vi "Host.vi"() -> ()   [LabVIEW 2022 SP3]
uses:
  <vilib>/FPGAPlugInAG/PXIe-7972R/niLvFpga_Open_PXIe-7972R.vi
  <vilib>/rvi/interface/common/dynamic/niFpgaDynamicAddResources.vi
  <vilib>/Utility/error.llb/Error Cluster From Error Code.vi
  <vilib>/rvi/errors/niLvFpgaAdjustHostInterfaceError.vi
  <vilib>/FPGAPlugInAG/Dynamic/niLvFpga_Close_Dynamic.vi
  <vilib>/rvi/interface/nirviOpenFPGA/nirviOpenFPGA.xnode
  FPGA Bitfiles/untitledproject1_FPGATarget_7972RFPGAVIfirst_8hhnNsn05bY.lvbitx
  <vilib>/rvi/interface/nirviMethod/nirviMethod.xnode
  <vilib>/rvi/interface/nirviReadWriteControl/nirviReadWriteControl.xnode
  <vilib>/rvi/interface/nirviCloseFPGA/nirviCloseFPGA.xnode
  <vilib>/FPGAPlugInAG/Dynamic/niLvFpga_ReadFifo_Dynamic.vi
  <vilib>/rvi/errors/niLvFpgaMergeErrorWithErrorCode.vi
  NiFpgaLv.dll
  <vilib>/rvi/interface/Simulation/niFpgaSimulationCallBeginRW.vi
panel:
  out "Genarated\nSignal":waveform(i16)(graph)
  in  "Number of Elements":u32
  in  "White Noise Amplitude":u16
  out "X":waveform(i16)(graph)
  in  "Sine Frequency":dbl
  in  "Add white noise?":bool
  in  "Signal Generator\nSelect":enum16{"Square", "Sawtooth", "Sine"}(ring)
  out "AI 1 - Filtered 2":waveform(dbl)(graph)
  in  "DMA FIFO Resolution":u32
  in  "Sawtooth Frequency":i16
  in  "Square Frequency":i16
  out "Y":waveform(i16)(graph)
  out "AI 1 - Raw":waveform(dbl)(graph)
  in  "stop":bool
  out "error out":errorcluster
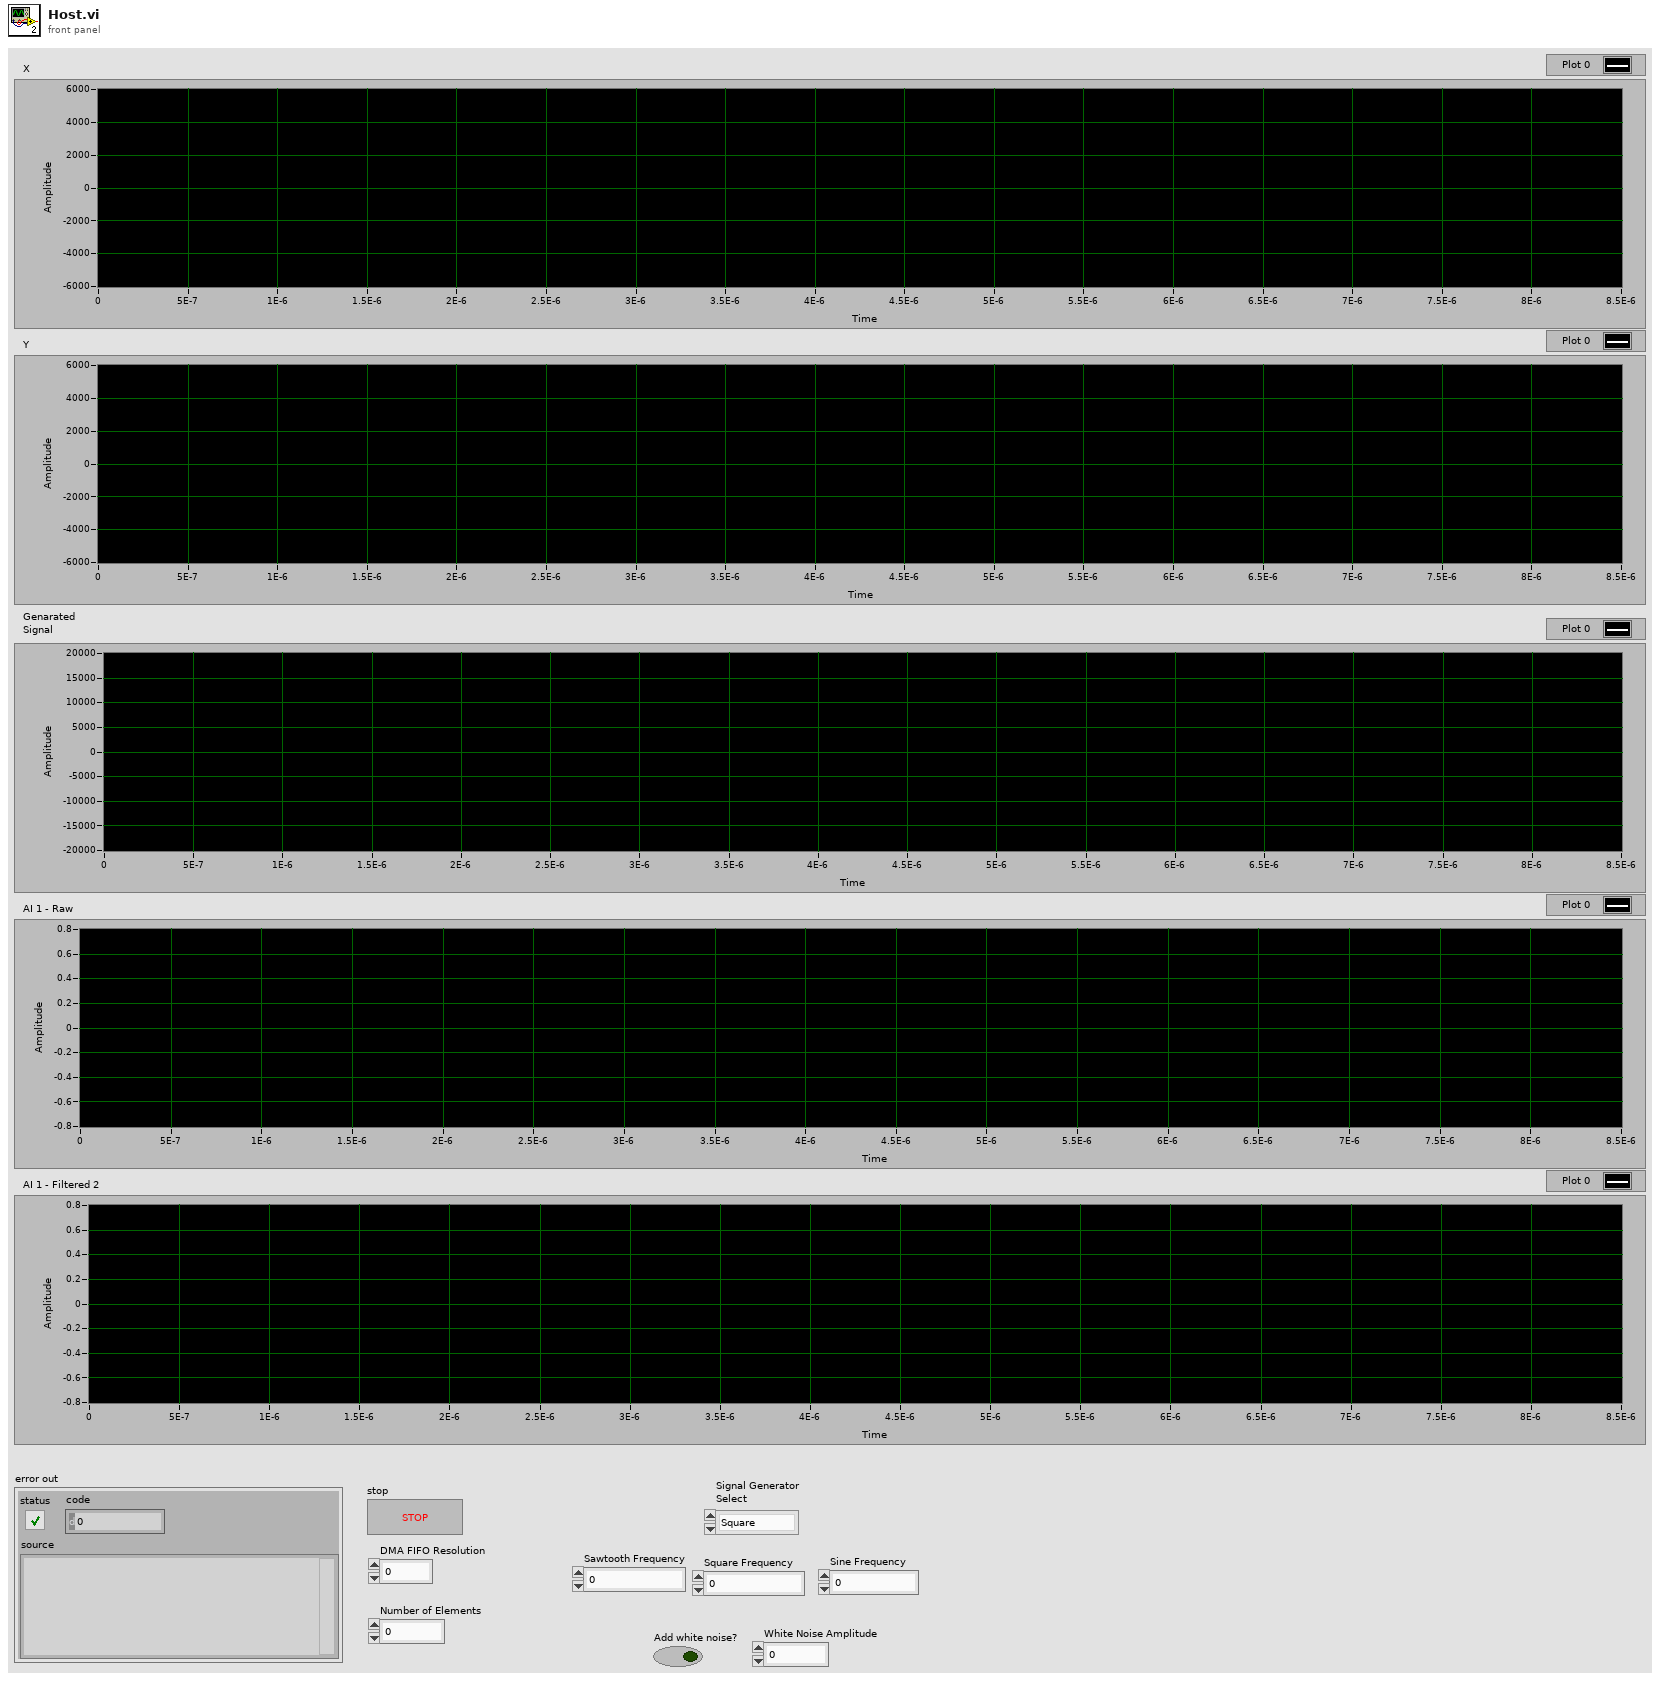
[diagram p1: front panel]
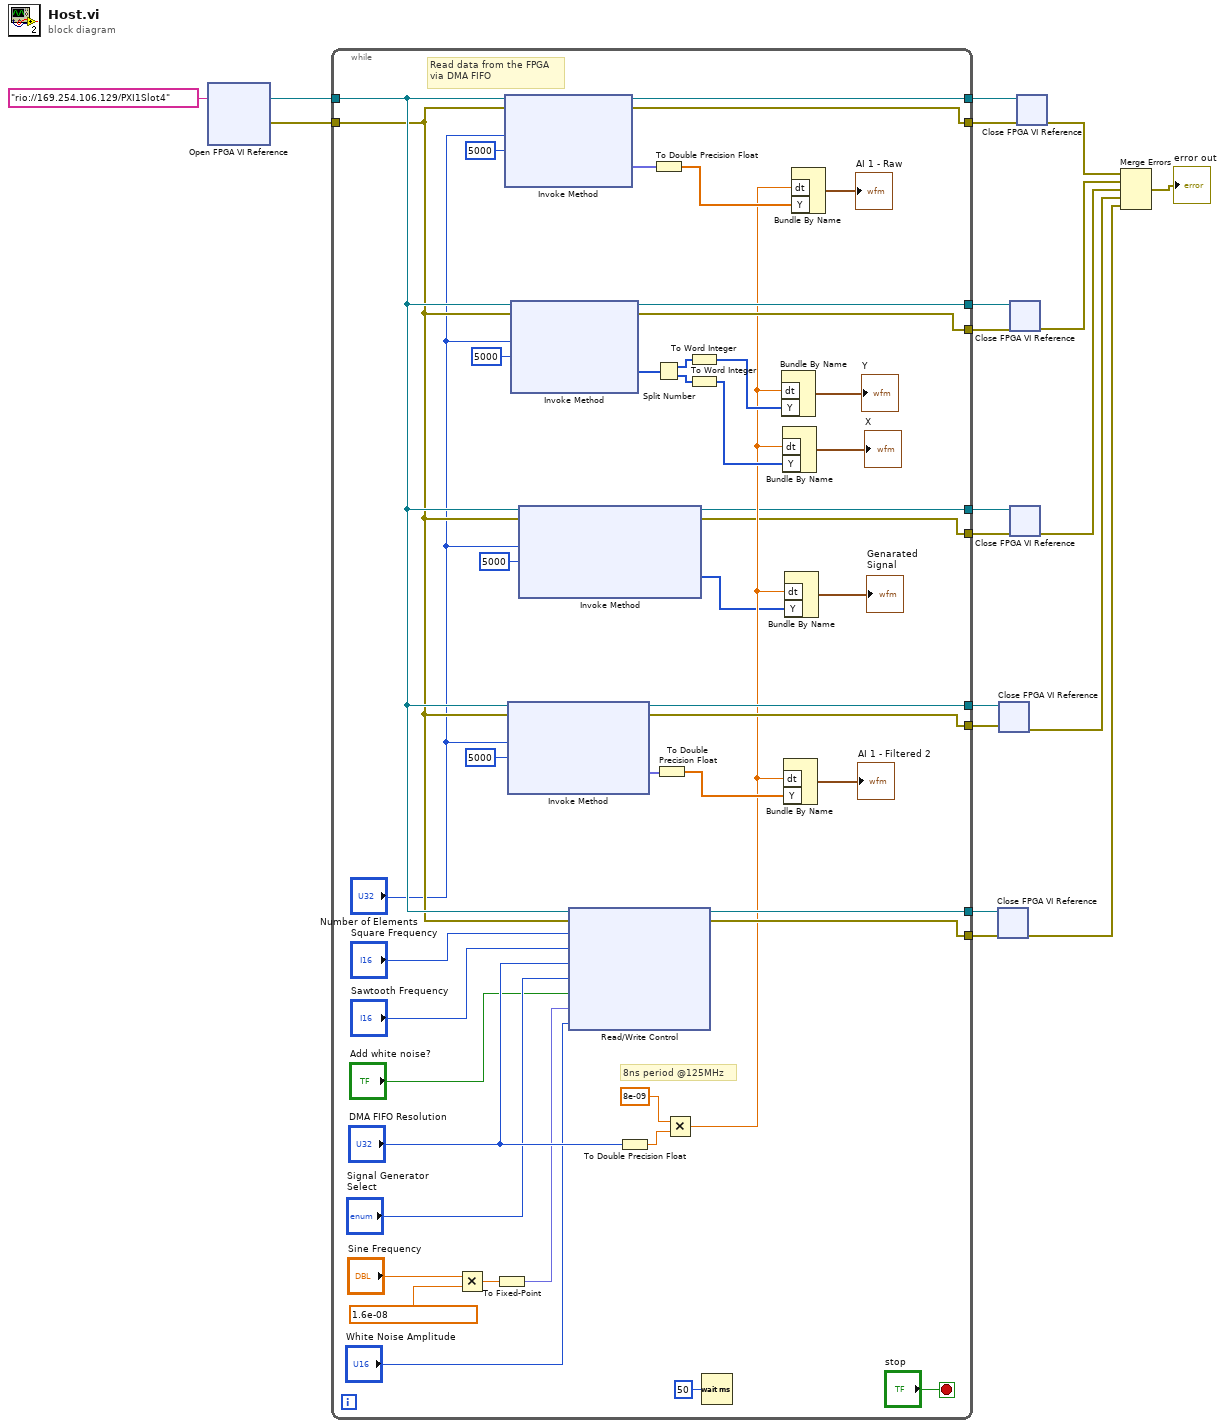
[diagram p0: block diagram]
diagram:
  n1 = xnode "Open FPGA VI Reference"("resource name"=tag "rio://169.254.106.129/PXI1Slot4") -> ("FPGA VI Reference Out"=w18:refnum<k20>, "error out"=w17:errorcluster)  [unwired: 1 in]
  n2 = while {
    tunnel: w18 -> [w27]
    tunnel: w17 -> [w26]
    tunnel: [w63] -> w16
    tunnel: [w60] -> w15
    tunnel: [w59] -> w12
    tunnel: [w57] -> w14
    tunnel: [w58] -> w10
    tunnel: [w30] -> w8
    tunnel: [w48] -> w7
    tunnel: [w47] -> w6
    tunnel: [w22] -> w3
    tunnel: [w21] -> w2
    stop <- "stop" stop-if-true
    # "Read data from the FPGA\nvia DMA FIFO"
    # "8ns period @125MHz"
    n3 = Multiply(x="Sine Frequency", y=1.6e-08 ("delta_t")) -> (x*y=w43:dbl)
    n4 = To Fixed-Point(number=w43) -> (fixed-point=w39:fxp<+/-,64,4>)  [unwired: 1 in]
    n5 = xnode "Invoke Method"("FPGA VI Reference In"=w27, "error in"=w26, "Number of Elements"="Number of Elements", "Timeout (ms)"=5000) -> ("FPGA VI Reference Out"=w63:refnum<k20>, "error out"=w59:errorcluster, "Data"=w62:fxp<+/-,25,2>[])  [unwired: 1 out]
    n6 = xnode "Invoke Method"("FPGA VI Reference In"=w27, "error in"=w26, "Number of Elements"="Number of Elements", "Timeout (ms)"=5000) -> ("FPGA VI Reference Out"=w48:refnum<k20>, "error out"=w47:errorcluster, "Data"=w50:fxp<+/-,25,2>[])  [unwired: 1 out]
    n7 = xnode "Invoke Method"("FPGA VI Reference In"=w27, "error in"=w26, "Number of Elements"="Number of Elements", "Timeout (ms)"=5000) -> ("FPGA VI Reference Out"=w57:refnum<k20>, "error out"=w58:errorcluster, "Data"=w37:u32[])  [unwired: 1 out]
    n8 = xnode "Invoke Method"("FPGA VI Reference In"=w27, "error in"=w26, "Number of Elements"="Number of Elements", "Timeout (ms)"=5000) -> ("FPGA VI Reference Out"=w22:refnum<k20>, "error out"=w21:errorcluster, "Data"=w23:i16[])  [unwired: 1 out]
    n9 = xnode "Read/Write Control"("FPGA VI Reference In"=w27, "error in"=w26, "Square Frequency"="Square Frequency", "Sawtooth Frequency"="Sawtooth Frequency", "DMA FIFO Resolution"="DMA FIFO Resolution", "Signal Generator Select"="Signal Generator\nSelect", "Add white noise?"="Add white noise?", "Sine delta_t"=w39, "White Noise Amplitude"="White Noise Amplitude") -> ("FPGA VI Reference Out"=w60:refnum<k20>, "error out"=w30:errorcluster)
    n10 = To Double Precision Float(number="DMA FIFO Resolution") -> (double precision float=w51:dbl)
    n11 = To Double Precision Float(number=w62) -> (double precision float=w42:dbl[])
    n12 = Split Number(x=w37) -> (hi(x)=w35:u16[], lo(x)=w33:u16[])
    n13 = To Double Precision Float(number=w50) -> (double precision float=w29:dbl[])
    n14 = Multiply(x=8e-09 ("dt"), y=w51) -> (x*y=w24:dbl)
    n15 = To Word Integer(number=w35) -> (16bit integer=w34:i16[])
    n16 = To Word Integer(number=w33) -> (16bit integer=w32:i16[])
    n17 = Wait (ms)(milliseconds to wait=u32 50) -> ()  [unwired: 1 out]
    n18 = Bundle By Name("dt"=w24, "Y"=w34) -> (→"Y":waveform(i16))  [unwired: 1 in]
    n19 = Bundle By Name("dt"=w24, "Y"=w32) -> (→"X":waveform(i16))  [unwired: 1 in]
    n20 = Bundle By Name("dt"=w24, "Y"=w29) -> (→"AI 1 - Filtered 2":waveform(dbl))  [unwired: 1 in]
    n21 = Bundle By Name("dt"=w24, "Y"=w23) -> (→"Genarated\nSignal":waveform(i16))  [unwired: 1 in]
    n22 = Bundle By Name("dt"=w24, "Y"=w42) -> (→"AI 1 - Raw":waveform(dbl))  [unwired: 1 in]
  }
  n23 = xnode "Close FPGA VI Reference"("FPGA VI Reference In"=w15, "error in"=w8) -> ("error out"=w4:errorcluster)
  n24 = xnode "Close FPGA VI Reference"("FPGA VI Reference In"=w7, "error in"=w6) -> ("error out"=w5:errorcluster)
  n25 = xnode "Close FPGA VI Reference"("FPGA VI Reference In"=w14, "error in"=w10) -> ("error out"=w9:errorcluster)
  n26 = xnode "Close FPGA VI Reference"("FPGA VI Reference In"=w3, "error in"=w2) -> ("error out"=w1:errorcluster)
  n27 = xnode "Close FPGA VI Reference"("FPGA VI Reference In"=w16, "error in"=w12) -> ("error out"=w11:errorcluster)
  n28 = Merge Errors(w11, w9, w1, w5, w4) -> (→"error out":errorcluster)
